vi "fg_event_to_sub.vi"(7 "fg_command":T4=enum."read", 8 "error in (no error)":errorcluster) -> (0 "error out":errorcluster, 2 "data":T3, 3 "to_sub":refnum<user-event>)   [LabVIEW 2015, in "lv-interface-sub-common.lvlib"]
uses:
  lv-interface-sub-common.lvlib
  _controls/fg_command.ctl
  _controls/event_to_sub_command.ctl
  _controls/interface_selection.ctl
  lv-interface-dom-nre/public/_controls/fg_command.ctl
  lv-interface-dom-nre/lv-interface-dom-nre.lvlib
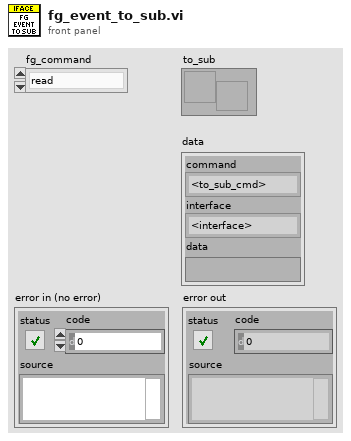
[diagram p1: front panel]
types:
  T1 = typedef "lv-interface-sub-common.lvlib/event_to_sub_command.ctl" = enum16{"<to_sub_cmd>", "die", "focus", "unfocus", "<null>"}
  T2 = typedef "lv-interface-sub-common.lvlib/interface_selection.ctl" = enum16{"<interface>", "sub_interface_1", "sub_interface_2", "<null>"}
  T3 = cluster{"command":T1, "interface":T2, "data":variant}
  T4 = typedef "lv-interface-sub-common.lvlib/fg_command.ctl" = enum16{"<fg_command>", "initialize", "read", "write", "shutdown", "<null>"}
  T5 = typedef "lv-interface-dom-nre.lvlib/fg_command.ctl" = enum16{"<fg_command>", "initialize", "read", "write", "shutdown", "<null>"}
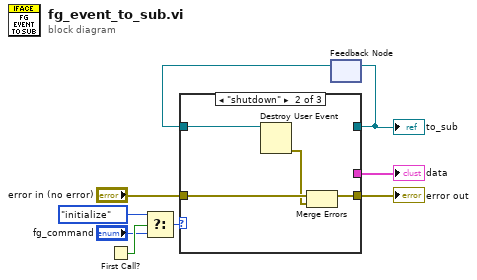
[diagram p0: block diagram]
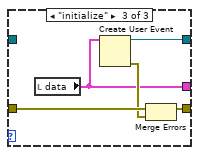
[diagram p3: hidden frame]
diagram:
  n1 = First Call?() -> (First Call?: T/F=w4:bool)
  n2 = Select(t=fg_command."initialize", s=w4, f="fg_command") -> (s? t:f=w1:T4)
  n3 = feedback #1() -> (w5:refnum<user-event>)  [unwired: 1 in]
  n4 = case shown="\"shutdown\"" w1 {
    tunnel: "error in (no error)" -> [w11 w15 w20]
    tunnel: [w10 _ w18] -> w6
    tunnel: [_ _ w17] -> w8
    tunnel: [w11 w14 w16] -> w7
    tunnel: w5 -> [w10 w12 _]
    frame "read", Default {
    }
    frame "shutdown" {
      n5 = Destroy User Event(user event=w12) -> (error out=w13:errorcluster)  [unwired: 1 in]
      n6 = Merge Errors(w15, w13) -> (w14:errorcluster)
    }
    frame "initialize" {
      n7 = local read "data"() -> (w17:T3)
      n8 = Create User Event(user event datatype=w17) -> (user event=w18:refnum<user-event>, error out=w19:errorcluster)  [unwired: 1 in]
      n9 = Merge Errors(w20, w19) -> (w16:errorcluster)
    }
  }
  "error out" <- w7
  "data" <- w8
  "to_sub" <- w6
  n10 = feedback-in #1(w6) -> ()
